vi "Do-Fft-Fpga-Top-Level-Multiple-Calls.vi"() -> ()   [LabVIEW 2014]
uses:
  <vilib>/FPGA/interface/niFpgaViExecutionMode.ctl
panel:
  out "Results (run 1)":csg[](array[numeric])
  out "FPGA VI Execution Mode":T1
  out "Comparison failed at\nindex:":i32=8
  out "Results Match!":bool
  out "Results Filename":string="data_16_1-results.txt"
  out "Expected Results (truncated)":csg[](array[numeric])
  out "size(s)":i32=16
  in  "SourceFileName":string="data_16_1.txt"
  out "Results (run 2)":csg[](array[numeric])
  out "error out":errorcluster
  out "Complex Data (in)":csg[](array[numeric])=[1.0+1.0i, 2.0+1.0i, 3.0+0.55i, 4.0+0.0i, 5.0+1.5i, 6.0+2.0i, 7.0+0.55i, 8.0+0.0i, 9.0+1.0i, 10.0+2.0i, 11.0+0.55i, 12.0+0.0i, 13.0+1.0i, 14.0+2.0i, 15.0+0.55i, 16.0+0.27i]
  in  "error in":errorcluster
  # "<===== 1 value does not match"
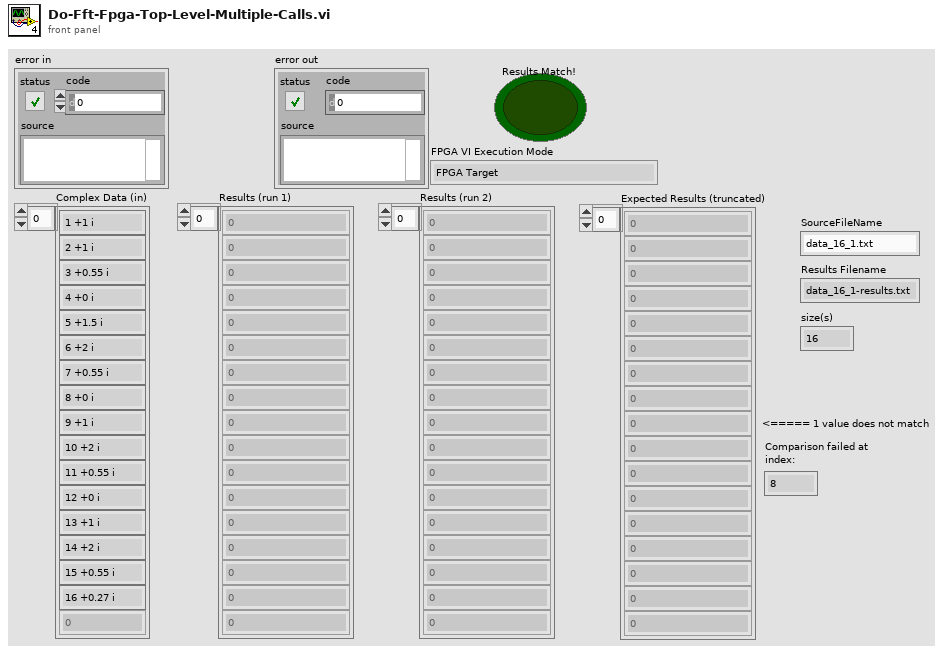
[diagram p1: front panel]
types:
  T1 = typedef "niFpgaViExecutionMode.ctl" = enum16{"FPGA Target", "Simulation (Simulated I/O)", "Simulation (Real I/O)", "Third-Party Simulation"}
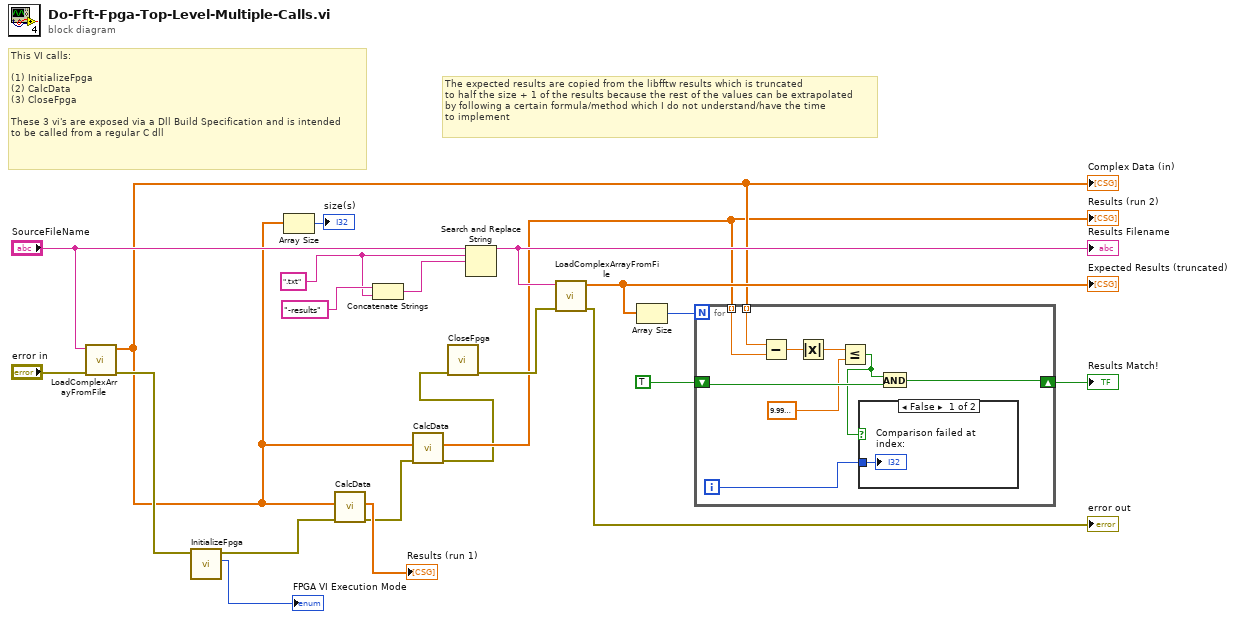
[diagram p0: block diagram]
diagram:
  w11 = ".txt" ("substring (\"\")")
  # "The expected results are copied from the libfftw results which is truncated\nto half the size + 1 of the results because the rest of the values can be extrapolated\nby following a certain formula/method which I do not understand/have the time\nto implement"
  # "This VI calls:\n\n(1) InitializeFpga\n(2) CalcData\n(3) CloseFpga\n\nThese 3 vi's are exposed via a Dll Build Specification and is intended\nto be called from a regular C dll"
  n1 = call "LoadComplexArrayFromFile.vi"("error in"="error in", "SourceFileName"="SourceFileName") -> ("error out"=w19:errorcluster, "Array"=w3:csg[])  [unwired: 8 in]
  "Complex Data (in)" <- w3
  n2 = call "InitializeFpga.vi"("error in"=w19) -> ("FPGA VI Execution Mode"=→"FPGA VI Execution Mode":T1, "error out"=w21:errorcluster)  [unwired: 9 in]
  n3 = Array Size(array=w3) -> (size(s)=→"size(s)":i32)
  n4 = call "CalcData.vi"("error in (no error)"=w21, "Complex Data (in)"=w3) -> ("error out"=w4:errorcluster, "Array out"=→"Results (run 1)":csg[])  [unwired: 8 in]
  n5 = Concatenate Strings("-results" ("replace string (\"\")"), w11) -> (w13:string)
  n6 = call "CalcData.vi"("error in (no error)"=w4, "Complex Data (in)"=w3) -> ("error out"=w1:errorcluster, "Array out"=w2:csg[])  [unwired: 8 in]
  "Results (run 2)" <- w2
  n7 = call "CloseFpga.vi"("error in"=w1) -> ("error out"=w15:errorcluster)  [unwired: 10 in]
  n8 = Search and Replace String(input string="SourceFileName", search string=w11, replace string=w13) -> (result string=w16:string)  [unwired: 5 in, 3 out]
  "Results Filename" <- w16
  n9 = call "LoadComplexArrayFromFile.vi"("error in"=w15, "SourceFileName"=w16) -> ("error out"=→"error out":errorcluster, "Array"=w10:csg[])  [unwired: 8 in]
  "Expected Results (truncated)" <- w10
  n10 = Array Size(array=w10) -> (size(s)=w9:i32)
  n11 = for {
    N: w9 -> [_]
    shift-right: [w30] -> w7
    shift-left: TRUE -> [w29]
    tunnel: w2 -> [w27] mode=indexing
    tunnel: w3 -> [w28] mode=indexing
    i -> [w22]
    n12 = Subtract(x=w28, y=w27) -> (x-y=w26:csg)
    n13 = Absolute Value(x=w26) -> (abs(x)=w25:sgl)
    n14 = Less Or Equal?(x=w25, y=sgl 1e-08) -> (x <= y?=w23:bool)
    n15 = case shown="False" w23 {
      tunnel: w22 -> [w31 _]
      frame False {
        "Comparison failed at\nindex:" <- w31
      }
      frame True {
      }
    }
    n16 = And(x=w23, y=w29) -> (x .and. y?=w30:bool)
  }
  "Results Match!" <- w7
